vi "Ensight_Format_Check.vi"(8 "error in":errorcluster, 11 "Input Number":dbl) -> (0 "error":errorcluster, 2 "Output field width":i32, 3 "Output string":string)   [LabVIEW 2022 SP3]
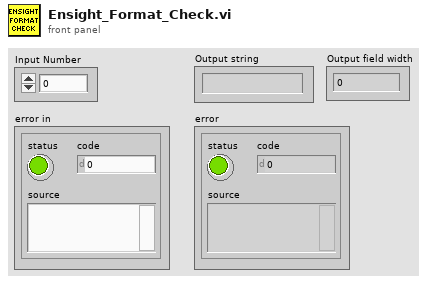
[diagram p1: front panel]
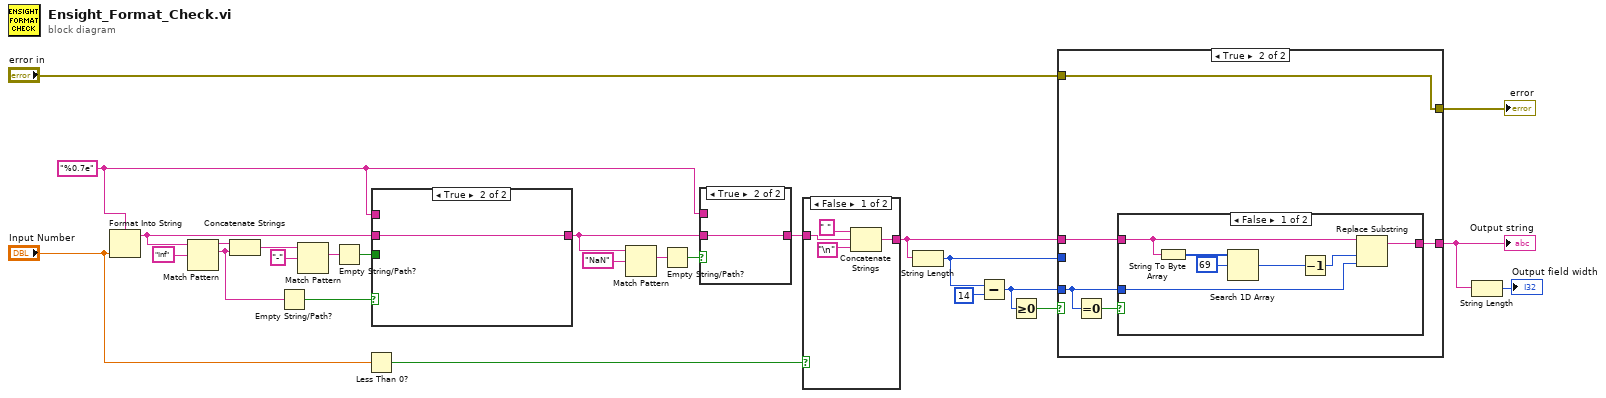
[diagram p0: block diagram]
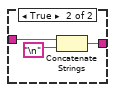
[diagram p2: hidden frame]
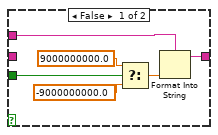
[diagram p3: hidden frame]
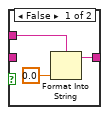
[diagram p4: hidden frame]
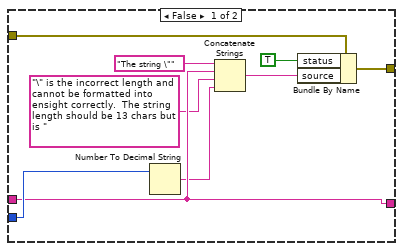
[diagram p5: hidden frame]
diagram:
  w9 = "%0.7e" ("format string")
  n1 = Format Into String(format string=w9, "Input Number") -> (resulting string=w10:string)  [unwired: 2 in, 1 out]
  n2 = Match Pattern(string=w10, regular expression="Inf") -> (before substring=w5:string, match substring=w1:string)  [unwired: 1 in, 2 out]
  n3 = Concatenate Strings(w5, w1) -> (w4:string)
  n4 = Empty String/Path?(string/path=w1) -> (empty?=w16:bool)
  n5 = Match Pattern(string=w4, regular expression="-") -> (match substring=w7:string)  [unwired: 1 in, 3 out]
  n6 = Empty String/Path?(string/path=w7) -> (empty?=w6:bool)
  n7 = Less Than 0?(x="Input Number") -> (x < 0?=w14:bool)
  n8 = case shown="True" w16 {
    tunnel: w10 -> [_ w33]
    tunnel: [w31 w33] -> w15
    tunnel: w9 -> [w32 _]
    tunnel: w6 -> [w30 _]
    frame False {
      n9 = Select(t=9000000000.0 ("input 1"), s=w30, f=-9000000000.0 ("input 1")) -> (s? t:f=w28:dbl)
      n10 = Format Into String(format string=w32, w28) -> (resulting string=w31:string)  [unwired: 2 in, 1 out]
    }
    frame True {
    }
  }
  n11 = Match Pattern(string=w15, regular expression="NaN") -> (match substring=w18:string)  [unwired: 1 in, 3 out]
  n12 = Empty String/Path?(string/path=w18) -> (empty?=w17:bool)
  n13 = case shown="True" w17 {
    tunnel: w15 -> [_ w37]
    tunnel: [w35 w37] -> w12
    tunnel: w9 -> [w36 _]
    frame False {
      n14 = Format Into String(format string=w36, 0.0 ("input 1")) -> (resulting string=w35:string)  [unwired: 2 in, 1 out]
    }
    frame True {
    }
  }
  n15 = case shown="False" w14 {
    tunnel: [w39 w43] -> w11
    tunnel: w12 -> [w40 w42]
    frame False {
      n16 = Concatenate Strings(" " ("string"), w40, "\n") -> (w39:string)
    }
    frame True {
      n17 = Concatenate Strings(w42, "\n") -> (w43:string)
    }
  }
  n18 = String Length(string=w11) -> (length=w20:i32)
  n19 = Subtract(x=w20, y=14) -> (x-y=w21:i32)
  n20 = Greater Or Equal To 0?(x=w21) -> (x >= 0?=w22:bool)
  n21 = case shown="True" w22 {
    tunnel: [w49 w58] -> w3
    tunnel: w11 -> [w49 w57]
    tunnel: w20 -> [w51 _]
    tunnel: [w45 w56] -> w25
    tunnel: "error in" -> [w53 w56]
    tunnel: w21 -> [_ w54]
    frame False {
      n22 = Number To Decimal String(number=w51) -> (decimal integer string=w47:string)  [unwired: 1 in]
      n23 = Concatenate Strings("The string \"" ("string"), w49, "\" is the incorrect length and cannot be formatted into ensight correctly.  The string length should be 13 chars but is " ("string"), w47) -> (w46:string)
      n24 = Bundle By Name(cluster=w53, "status"=TRUE, "source"=w46) -> (w45:errorcluster)
    }
    frame True {
      n25 = Equal To 0?(x=w54) -> (x = 0?=w55:bool)
      n26 = case shown="False" w55 {
        tunnel: [w65 w66] -> w58
        tunnel: w57 -> [w60 w66]
        tunnel: w54 -> [w59 _]
        frame False {
          n27 = String To Byte Array(string=w60) -> (unsigned byte array=w63:u8[])
          n28 = Search 1D Array(1D array=w63, element=u8 69) -> (index of element=w62:i32)  [unwired: 1 in]
          n29 = Decrement(x=w62) -> (x-1=w61:i32)
          n30 = Replace Substring(2:w59, 3:w61, 5:w60) -> (1:w65:string)  [unwired: 1 in, 1 out]
        }
        frame True {
        }
      }
    }
  }
  "Output string" <- w3
  "error" <- w25
  n31 = String Length(string=w3) -> (length=→"Output field width":i32)
